vi "Close Sample Container Connections.vi"(8 "error in (no error)":errorcluster, 11 "Container in":T1) -> (0 "error out":errorcluster, 3 "Container out":T1)   [LabVIEW 2015]
uses:
  Controls/Sample Container.ctl
  Sample/Sample.lvclass
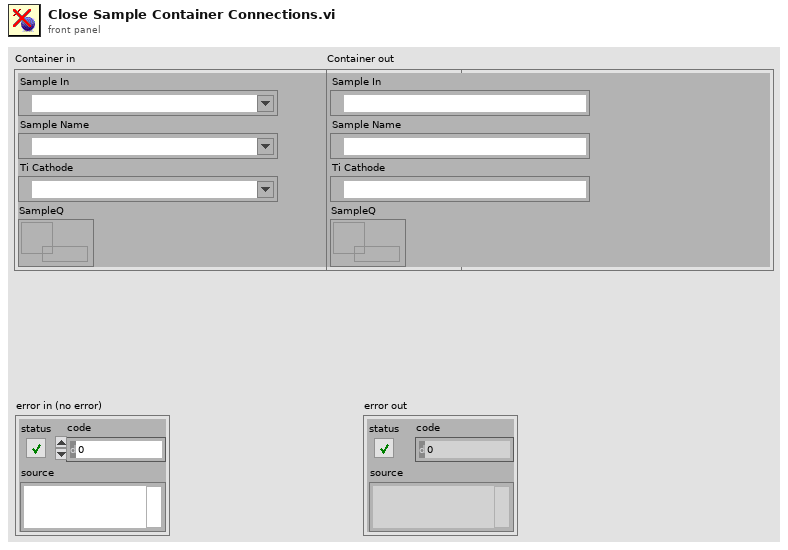
[diagram p1: front panel]
types:
  T1 = typedef "Sample Container.ctl" = cluster{"Sample In":refnum<k21>, "Sample Name":refnum<k21>, "Ti Cathode":refnum<k21>, "SampleQ":refnum<queue>}
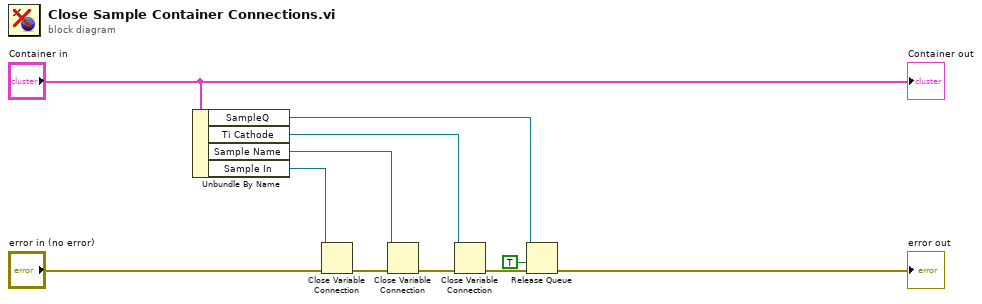
[diagram p0: block diagram]
diagram:
  n1 = Unbundle By Name("Container in") -> ("SampleQ"=w2:refnum<queue>, "Ti Cathode"=w7:refnum<k21>, "Sample Name"=w8:refnum<k21>, "Sample In"=w9:refnum<k21>)
  n2 = Close Variable Connection(8:"error in (no error)", 11:w9) -> (0:w6:errorcluster)
  n3 = Close Variable Connection(8:w6, 11:w8) -> (0:w5:errorcluster)
  n4 = Close Variable Connection(8:w5, 11:w7) -> (0:w4:errorcluster)
  n5 = Release Queue(queue=w2, force destroy? (F)=TRUE, error in (no error)=w4) -> (error out=→"error out":errorcluster)  [unwired: 2 out]
  "Container out" <- "Container in"
